vi "osc_acquire.vi"() -> ()   [LabVIEW 2015]
doc: "This example shows how to use autosetup and acquire a waveform on a single channel for acquiring waveforms in a loop until stopped by user."
uses:
  osc_channel.ctl
  osc_stats.ctl
  Global.vi
  oskar_tools/oskar_tools.lvlib
  daq_simulate/daq_simulate.lvlib
panel:
  out "SQUID":string="3"
  in  "stop":bool
  in  "Tab Control":T1(tab)
  out "Saving":bool
  out "Waveform Data":waveform(dbl)[](graph)=[{"t0"=timestamp(0 s since 1904-01-01), "dt"=6e-09, "Y"=array[1000 elements]}, {"t0"=timestamp(0 s since 1904-01-01), "dt"=6e-09, "Y"=array[1000 elements]}]
  in  "Points":i32=1000
  out "dt":dbl=6e-09 format="%#_2e"
  out "Repeat":u32=18
  out "Scope":cluster{"Manufacturer":string, "Model":string}
  in  "record stats.":bool[](array[boolean])=[TRUE, FALSE]
  out "Statistics":T2[](array[typedef])
  in  "Channels":T3[](array[typedef])=[{"channel name"="CHANNEL1", "probe attenuation"=1.0, "vertical offset"=0.0, "vertical range"=10.0, "vertical coupling"=1, "input impedance"=50.0}, {"channel name"="CHANNEL2", "probe attenuation"=1.0, "vertical offset"=0.0, "vertical range"=1.0, "vertical coupling"=1, "input impedance"=50.0}] caption="Settings" {"input impedance" format="%#_13g"; "vertical coupling" items=["AC", "DC", "GND"]; "vertical range" format="%.3f"; "vertical offset" format="%.3f"; "probe attenuation" format="%.3f"}
  in  "wait (ms)":u32=500
  in  "Bin size":i16=1
  in  "sample":dbl=6e-06
  in  "amplitude":dbl=1.0 format="%#_13g"
  in  "noise":dbl=0.1 format="%#_13g"
  in  "frequency":dbl=1000000.0 format="%#_13g"
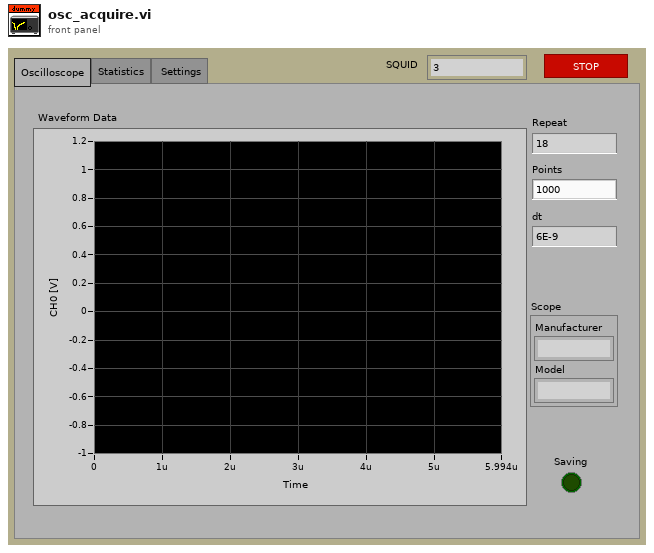
[diagram p1: front panel]
types:
  T1 = enum32{"Oscilloscope", "Statistics", " Settings"}
  T2 = typedef "osc_stats.ctl" = cluster{"min":dbl, "t_min":dbl, "max":dbl, "t_max":dbl, "range":dbl, "mean":dbl, "stdev":dbl}
  T3 = typedef "osc_channel.ctl" = cluster{"channel name":string, "probe attenuation":dbl, "vertical offset":dbl, "vertical range":dbl, "vertical coupling":i32, "input impedance":dbl}
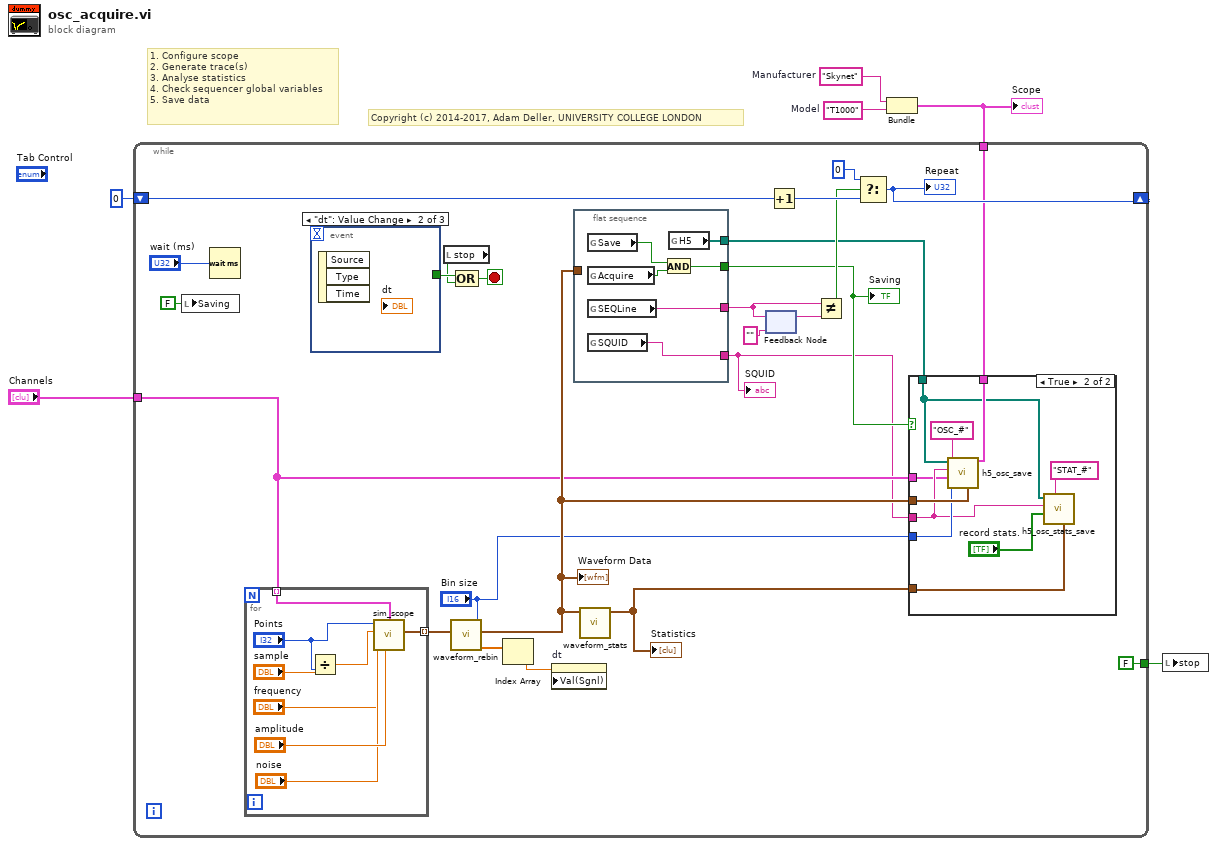
[diagram p0: block diagram]
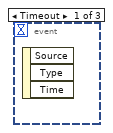
[diagram p3: hidden frame]
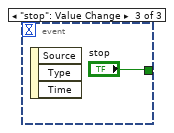
[diagram p4: hidden frame]
diagram:
  w2 = "T1000"  # Model
  w1 = "Skynet"  # Manufacturer
  # "Copyright (c) 2014-2017, Adam Deller, UNIVERSITY COLLEGE LONDON"
  # "1. Configure scope\n2. Generate trace(s)\n3. Analyse statistics\n4. Check sequencer global variables\n5. Save data"
  n1 = Bundle("Manufacturer"=w1, "Model"=w2) -> (w3:cluster{"Manufacturer":string, "Model":string})  [unwired: 1 in]
  "Scope" <- w3
  n2 = while {
    shift-right: [w28] -> _
    shift-left: u32 0 ("millisecond multiple") -> [w29]
    tunnel: [FALSE ("stop")] -> w5
    tunnel: "Channels" -> [w19]
    tunnel: w3 -> [w11]
    stop <- w30 stop-if-true
    n3 = local write "Saving"(FALSE ("Saving")) -> ()
    n4 = Wait (ms)(milliseconds to wait="wait (ms)") -> ()  [unwired: 1 out]
    n5 = for {
      tunnel: [w55] -> w22 mode=indexing
      tunnel: w19 -> [w56] mode=indexing
      n6 = Divide(x="sample", y="Points") -> (x/y=w54:dbl)
      n7 = call "sim_scope.vi"("amplitude"="amplitude", "CHAN"=w56, "frequency"="frequency", "noise"="noise", "dt"=w54, "Points"="Points") -> ("output waveform"=w55:waveform(dbl))  [unwired: 5 in]
    }
    n8 = event shown="[1] \"dt\": Value Change" {
      selector: _ -> [_ _ _]
      dyn-events: _ -> [_ _ _]
      timeout: _ -> [_ _ _]
      tunnel: [_ _ "stop"] -> w26
      event Timeout {
        n9 = event-data() -> ()  [unwired: 1 in, 3 out]
      }
      event "dt": Value Change {
        n10 = event-data() -> ()  [unwired: 1 in, 3 out]
      }
      event "stop": Value Change {
        n11 = event-data() -> ()  [unwired: 1 in, 3 out]
      }
    }
    n12 = local read "stop"() -> (w25:bool)
    n13 = call "waveform_rebin.vi"("Bin size"="Bin size", "Waveform Data IN"=w22) -> ("dt"=w21:dbl[], "Waveform Data OUT"=w23:waveform(dbl)[])  [unwired: 6 in, 1 out]
    "Waveform Data" <- w23
    n14 = Compound Arithmetic op=OR(w26, w25) -> (w30:bool)
    n15 = Index Array(array=w21) -> (element=w10:dbl)  [unwired: 1 in]
    n16 = property on="dt" class="DigNum (strict)"("Val(Sgnl)"=w10) -> ()  [unwired: 2 in, 2 out]
    n17 = flat-sequence {
      tunnel: w23 -> [_]
      tunnel: [w35] -> w14
      tunnel: [w34] -> w8
      tunnel: [w32] -> w7
      tunnel: [w33] -> w12
      frame #0 {
        n18 = global read "Global.vi" "Save"() -> (w36:bool)
        n19 = global read "Global.vi" "Acquire"() -> (w37:bool)
        n20 = global read "Global.vi" "SEQLine"() -> (w34:string)
        n21 = global read "Global.vi" "SQUID"() -> (w32:string)
        n22 = And(x=w36, y=w37) -> (x .and. y?=w35:bool)
        n23 = global read "Global.vi" "H5"() -> (w33:path[])
      }
    }
    n24 = call "waveform_stats.vi"("Waveform Data"=w23) -> ("stats"=w13:T2[])  [unwired: 7 in]
    "Statistics" <- w13
    n25 = feedback #1("" ("Seq")) -> (w9:string)
    n26 = feedback-in #1(w8) -> ()
    n27 = Increment(x=w29) -> (x+1=w17:u32)
    n28 = Not Equal?(x=w8, y=w9) -> (x != y?=w16:bool)
    n29 = Select(t=u32 0, s=w16, f=w17) -> (s? t:f=w28:u32)
    "Repeat" <- w28
    n30 = case shown="True" w14 {
      tunnel: w23 -> [_ w47]
      tunnel: w19 -> [_ w38]
      tunnel: w7 -> [_ w43]
      tunnel: "Bin size" -> [_ w44]
      tunnel: w13 -> [_ w39]
      tunnel: w12 -> [_ w42]
      tunnel: w11 -> [_ w45]
      frame False {
      }
      frame True {
        n31 = call "h5_osc_save.vi"("Waveform Data"=w47, "Scope"=w45, "TYPE"="OSC_#", "Bin size"=w44, "Settings"=w38, "SQUID"=w43, "H5"=w42) -> ()  [unwired: 4 in, 1 out]
        n32 = call "h5_osc_stats_save.vi"("stats"=w39, "TYPE"="STAT_#", "record stats."="record stats.", "SQUID"=w43, "H5"=w42) -> ()  [unwired: 6 in, 1 out]
      }
    }
    "Saving" <- w14
    "SQUID" <- w7
  }
  n33 = local write "stop"(w5) -> ()
